vi "Panel-FringeProcessor-4.vi"() -> ()   [LabVIEW 2009]
uses:
  <vilib>/Analysis/4window.llb/windowTd.ctl
  <vilib>/measure/maspectr.llb/FFT Power Spectral Density for 1 Chan.vi
  <vilib>/measure/madcrms.llb/Basic Averaged DC-RMS for 1 Chan.vi
  <vilib>/measure/NI_MAPro.lvlib
  <vilib>/Analysis/NI_AALPro.lvlib
panel:
  in  "Spots / Full":bool
  out "Total flux":dbl[unit]
  out "Spot intensities":T1(graph)
  out "averaging done":bool
  in  "restart averaging (F)":bool
  in  "averaging parameters":T2={"averaging mode"=enum."No averaging", "weighting mode"=enum."Exponential", "number of averages"=10} {"number of averages" min=1}
  out "PSD":cluster{"f0":dbl, "df":dbl, "magnitude":dbl[]}(graph)
  out "S Polarization":waveform(dbl)(graph)
  out "P polarization (1-2)/(1+2)":waveform(dbl)(graph)
  in  "stop":bool
  out "Flux":i32[][](graph)
  out "Intensity Graph":i32[][](graph)
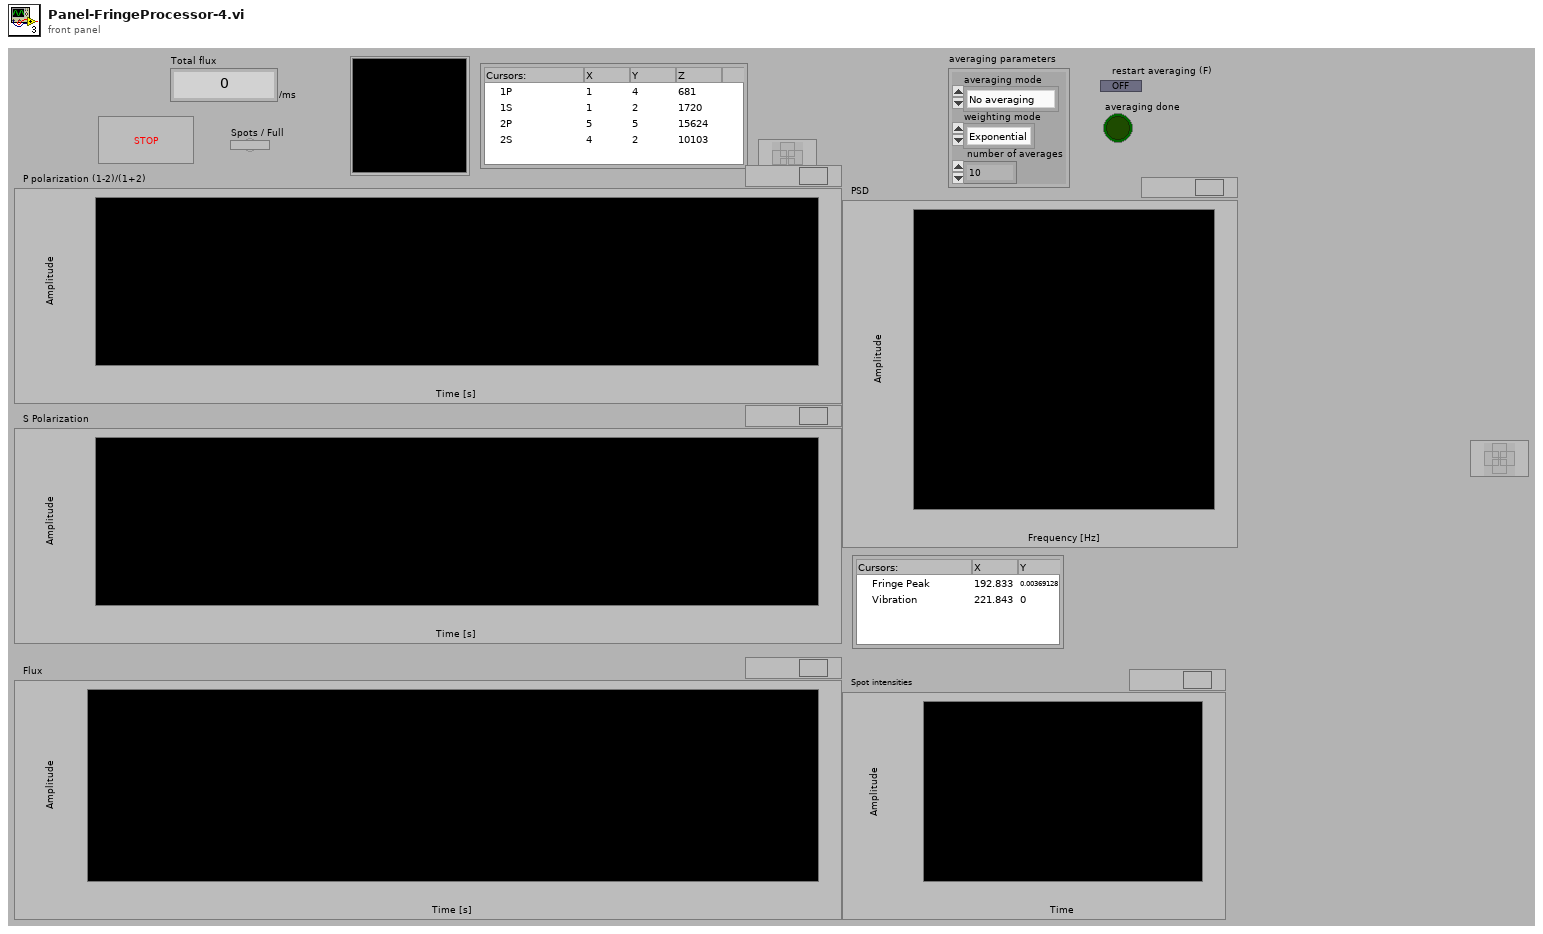
[diagram p1: front panel]
types:
  T1 = cluster{"[0]":i32, "[1]":i32, "[2]":i32, "[3]":i32, "[4]":i32, "[5]":i32, "[6]":i32, "[7]":i32, "[8]":i32}
  T2 = cluster{"averaging mode":enum16{"No averaging", "Vector averaging", "RMS averaging", "Peak hold"}, "weighting mode":enum16{"Linear", "Exponential"}, "number of averages":u32}
  T3 = typedef "NI_AALPro.lvlib/windowTd.ctl" = u32
  T4 = typedef "NICMOS.DATA.ctl" = cluster{"DATA":i32[][][], "INDEX":i32}
  T5 = typedef "NICMOS.READOUT.ctl" = cluster{"Readout":i32, "Deglitch":i32, "Framerate":dbl[unit], "Bank":i32}
  T6 = typedef "LVPointDoubleTypeDef.ctl" = cluster{"Cursor X":dbl, "Cursor Y":dbl}
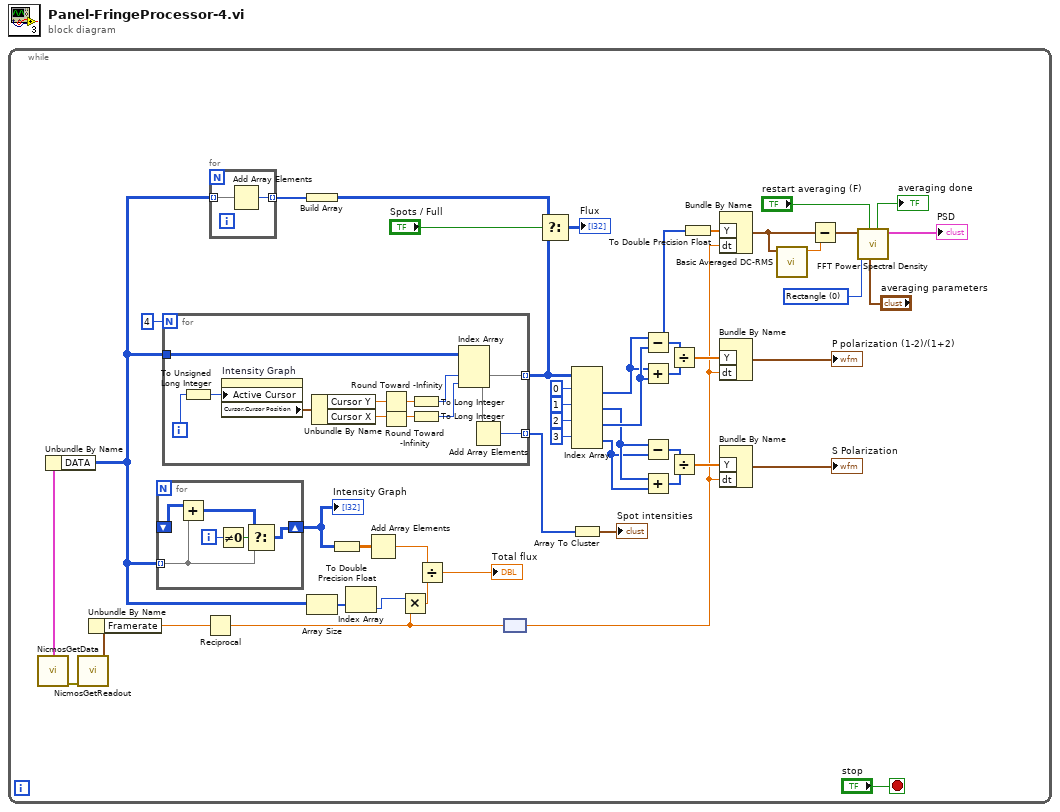
[diagram p0: block diagram]
diagram:
  n1 = while {
    stop <- "stop" stop-if-true
    w22 = T3 0 items=["Rectangle"=0, "Hanning"=1, "Hamming"=2, "Blackman-Harris"=3, "Exact Blackman"=4, "Blackman"=5, "Flat Top"=6, "4 Term B-Harris "=7, "7 Term B-Harris"=8, "Low Sidelobe"=9, "Blackman Nuttall"=11, "Triangle"=30, "Bartlett-Hanning"=31, "Bohman"=32, "Parzen"=33, "Welch"=34, "Kaiser"=60, "Dolph-Chebyshev"=61, "Gaussian"=62] ("window")
    n2 = call "NicmosGetData.vi"() -> ("DATA"=w48:T4, "error out"=w35:errorcluster)  [unwired: 8 in]
    n3 = Unbundle By Name(w48) -> ("DATA"=w6:i32[][][])
    n4 = call "NicmosGetReadout.vi"("error in (no error)"=w35) -> ("READOUT out"=w34:T5)  [unwired: 7 in, 1 out]
    n5 = Unbundle By Name(w34) -> ("Framerate"=w9:dbl[unit])
    n6 = for {
      tunnel: w6 -> [w66] mode=indexing
      shift-right: [w64] -> w17
      shift-left: _ -> [w63]
      i -> [w68]
      n7 = Add(x=w63, y=w66) -> (x+y=w65:i32[][])
      n8 = Not Equal To 0?(x=w68) -> (x != 0?=w67:bool)
      n9 = Select(t=w65, s=w67, f=w66) -> (s? t:f=w64:i32[][])
    }
    "Intensity Graph" <- w17
    n10 = for {
      N: 4 -> [_]
      tunnel: w6 -> [w58]
      tunnel: [w52] -> w3 mode=indexing
      tunnel: [w51] -> w21 mode=indexing
      i -> [w55]
      n11 = To Unsigned Long Integer(number=w55) -> (unsigned 32bit integer=w54:u32)
      n12 = property on="Intensity Graph" class="IntGraph (strict)"("Active Cursor"=w54) -> ("Cursor.Cursor Position"=w53:T6)  [unwired: 2 in, 2 out]
      n13 = Unbundle By Name(w53) -> ("Cursor Y"=w62:dbl, "Cursor X"=w61:dbl)
      n14 = Round Toward -Infinity(1:w62) -> (0:w60:dbl)
      n15 = Round Toward -Infinity(1:w61) -> (0:w59:dbl)
      n16 = To Long Integer(number=w60) -> (32bit integer=w57:i32)
      n17 = To Long Integer(number=w59) -> (32bit integer=w56:i32)
      n18 = Index Array(array=w58, index (dim 1)=w57, index (dim 2)=w56) -> (element=w52:i32[])  [unwired: 1 in]
      n19 = Add Array Elements(numeric array=w52) -> (sum=w51:i32)
    }
    n20 = Reciprocal(x=w9) -> (1/x=w11:dbl[unit])
    n21 = for {
      tunnel: w6 -> [w50] mode=indexing
      tunnel: [w49] -> w5 mode=indexing
      n22 = Add Array Elements(numeric array=w50) -> (sum=w49:i32)
    }
    n23 = Build Array(w5) -> (w4:i32[][])
    n24 = Array Size(array=w6) -> (size(s)=w14:i32[])
    n25 = To Double Precision Float(number=w17) -> (double precision float=w16:dbl[][])
    n26 = Index Array(array=w14) -> (element=w13:i32)  [unwired: 1 in]
    n27 = Add Array Elements(numeric array=w16) -> (sum=w15:dbl)
    n28 = Multiply(x=w13, y=w11) -> (x*y=w12:dbl[unit])
    n29 = Divide(x=w15, y=w12) -> (x/y=→"Total flux":dbl[unit])
    n30 = node(w11) -> (w10:dbl)
    n31 = Select(t=w4, s="Spots / Full", f=w3) -> (s? t:f=→"Flux":i32[][])
    n32 = Index Array(array=w3, index (row) #1=0 ("index (row)"), index (row) #2=1 ("index (row)"), index (row) #3=2 ("index (row)"), index (row) #4=3 ("index (row)")) -> (element #1=w7:i32[], element #2=w39:i32[], element #3=w41:i32[], element #4=w36:i32[])  [unwired: 4 in]
    n33 = Array To Cluster(array=w21) -> (cluster=→"Spot intensities":T1)
    n34 = Subtract(x=w7, y=w41) -> (x-y=w19:i32[])
    n35 = Add(x=w7, y=w41) -> (x+y=w40:i32[])
    n36 = Subtract(x=w39, y=w36) -> (x-y=w38:i32[])
    n37 = Add(x=w39, y=w36) -> (x+y=w37:i32[])
    n38 = Divide(x=w19, y=w40) -> (x/y=w31:dbl[])
    n39 = Divide(x=w38, y=w37) -> (x/y=w33:dbl[])
    n40 = To Double Precision Float(number=w19) -> (double precision float=w29:dbl[])
    n41 = Bundle By Name("Y"=w29, "dt"=w10) -> (w27:waveform(dbl))  [unwired: 1 in]
    n42 = Bundle By Name("Y"=w31, "dt"=w10) -> (→"P polarization (1-2)/(1+2)":waveform(dbl))  [unwired: 1 in]
    n43 = Bundle By Name("Y"=w33, "dt"=w10) -> (→"S Polarization":waveform(dbl))  [unwired: 1 in]
    n44 = call-poly <vilib>:"Basic Averaged DC-RMS.vi"("signal in"=w27) -> ("DC value"=w18:dbl)  [unwired: 7 in, 3 out]
    n45 = Subtract(x=w27, y=w18) -> (x-y=w26:waveform(dbl))
    n46 = call-poly <vilib>:"FFT Power Spectral Density.vi"("averaging parameters"="averaging parameters", "restart averaging (F)"="restart averaging (F)", "window"=w22, "time signal"=w26) -> ("power spectral density"=→"PSD":cluster{"f0":dbl, "df":dbl, "magnitude":dbl[]}, "averaging done"=→"averaging done":bool)  [unwired: 4 in, 2 out]
  }
